vi "ShooterB Test.vi"(0 "Shooter":dbl, 1 "Encoder":dbl, 2 "GetMotorOut":dbl) -> (3 "ToMotor":dbl, 4 "EncoderRPS 2":dbl, 5 "CurentSpeed":dbl, 6 "SpeedWanted":dbl)   [LabVIEW 2011]
uses:
  RobotBetImunim/Robot Global Data.vi
panel:
  out "Waveform Chart 2":dbl(graph)
  out "Waveform Chart":dbl(graph)
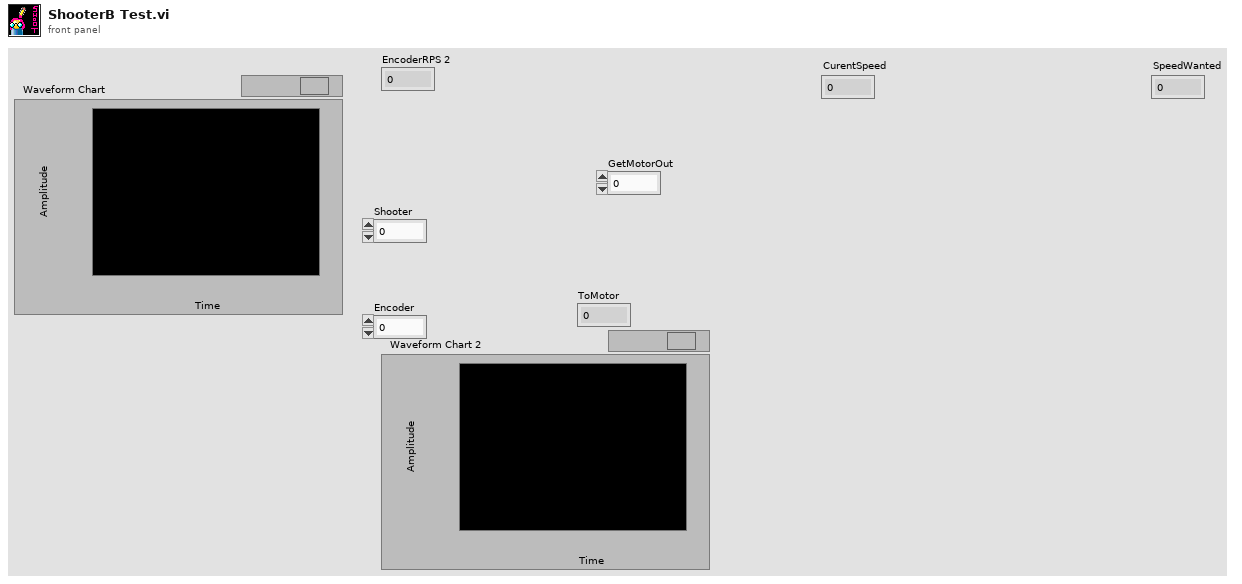
[diagram p1: front panel]
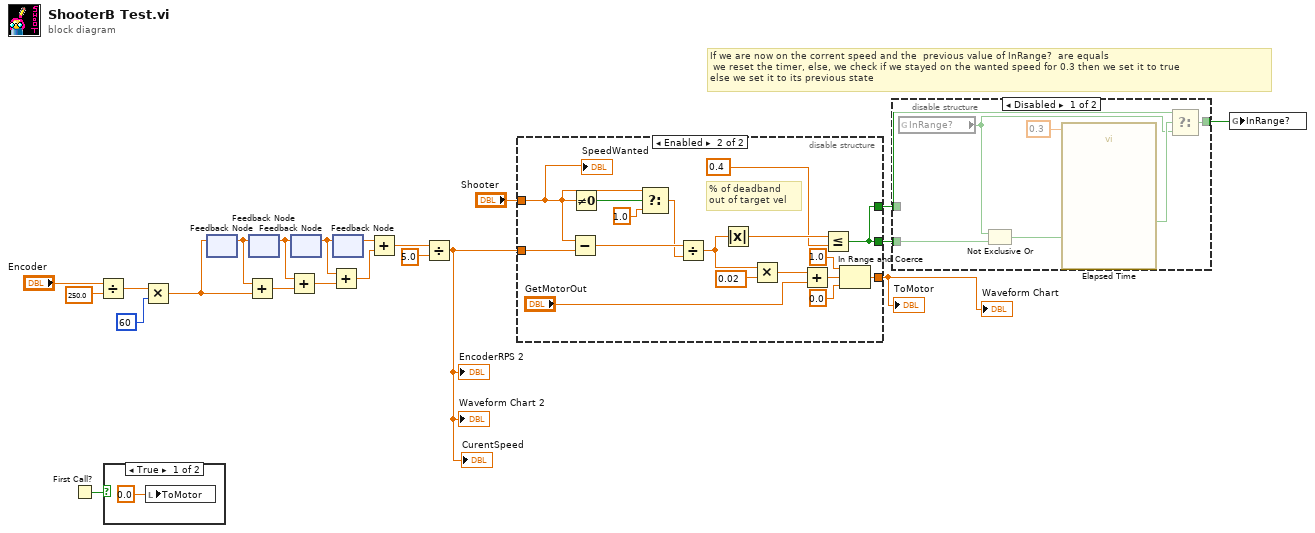
[diagram p0: block diagram]
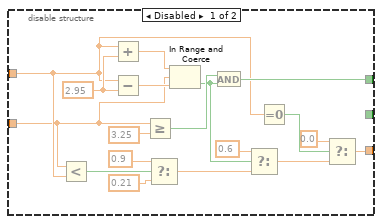
[diagram p4: hidden frame]
diagram:
  # "If we are now on the corrent speed and the  previous value of InRange?  are equals\n we reset the timer, else, we check if we stayed on the wanted speed for 0.3 then we set it to true\nelse we set it to its previous state"
  n1 = First Call?() -> (First Call?: T/F=w8:bool)
  n2 = Divide(x="Encoder", y=250.0) -> (x/y=w4:dbl)
  n3 = case shown="True" w8 {
    frame True {
      n4 = local write "ToMotor"(0.0 ("ToMotor")) -> ()
    }
    frame False {
    }
  }
  n5 = Multiply(x=w4, y=60) -> (x*y=w3:dbl)
  n6 = feedback #1() -> (w14:dbl)  [unwired: 1 in]
  n7 = feedback-in #1(w3) -> ()
  n8 = Add(x=w14, y=w3) -> (x+y=w13:dbl)
  n9 = feedback #2() -> (w18:dbl)  [unwired: 1 in]
  n10 = feedback-in #2(w14) -> ()
  n11 = Add(x=w18, y=w13) -> (x+y=w19:dbl)
  n12 = feedback #3() -> (w16:dbl)  [unwired: 1 in]
  n13 = feedback-in #3(w18) -> ()
  n14 = Add(x=w16, y=w19) -> (x+y=w17:dbl)
  n15 = feedback #4() -> (w15:dbl)  [unwired: 1 in]
  n16 = feedback-in #4(w16) -> ()
  n17 = Add(x=w15, y=w17) -> (x+y=w20:dbl)
  n18 = Divide(x=w20, y=5.0) -> (x/y=w1:dbl)
  "EncoderRPS 2" <- w1
  "Waveform Chart 2" <- w1
  "CurentSpeed" <- w1
  n19 = disable-structure shown="Enabled" {
    disable-tunnel: [w30 w44] -> w10
    disable-tunnel: [w27 w46] -> w6
    disable-tunnel: "Shooter" -> [w24 w41]
    disable-tunnel: w1 -> [w23 w57]
    disable-tunnel: [_ w46] -> w7
    frame Disabled {
      w39 = 2.95
      n20 = Less?(x=w23, y=w24) -> (x < y?=w25:bool)
      n21 = Add(x=w24, y=w39) -> (x+y=w38:dbl)
      n22 = Subtract(x=w24, y=w39) -> (x-y=w37:dbl)
      n23 = Greater Or Equal?(x=w23, y=3.25) -> (x >= y?=w28:bool)
      n24 = Select(t=0.9, s=w25, f=0.21) -> (s? t:f=w35:dbl)
      n25 = In Range and Coerce(upper limit=w38, x=w23, lower limit=w37) -> (In Range?=w26:bool)  [unwired: 1 out]
      n26 = And(x=w28, y=w26) -> (x .and. y?=w27:bool)
      n27 = Select(t=0.6, s=w26, f=w35) -> (s? t:f=w32:dbl)
      n28 = Equal To 0?(x=w24) -> (x = 0?=w31:bool)
      n29 = Select(t=0.0, s=w31, f=w32) -> (s? t:f=w30:dbl)
    }
    frame Enabled {
      # "% of deadband\nout of target vel"
      n30 = Subtract(x=w41, y=w57) -> (x-y=w54:dbl)
      n31 = Not Equal To 0?(x=w41) -> (x != 0?=w52:bool)
      n32 = Select(t=w41, s=w52, f=1.0) -> (s? t:f=w51:dbl)
      n33 = Divide(x=w54, y=w51) -> (x/y=w49:dbl)
      n34 = Absolute Value(x=w49) -> (abs(x)=w48:dbl)
      n35 = Multiply(x=w49, y=0.02) -> (x*y=w53:dbl)
      n36 = Add(x=w53, y="GetMotorOut") -> (x+y=w55:dbl)
      n37 = Less Or Equal?(x=w48, y=0.4) -> (x <= y?=w46:bool)
      n38 = In Range and Coerce(upper limit=1.0, x=w55, lower limit=0.0) -> (coerced(x)=w44:dbl)  [unwired: 1 out]
      "SpeedWanted" <- w41
    }
  }
  "ToMotor" <- w10
  "Waveform Chart" <- w10
  n39 = disable-structure shown="Disabled" {
    disable-tunnel: w7 -> [w64 _]
    disable-tunnel: w6 -> [w60 w65]
    disable-tunnel: [w59 w65] -> w5
    frame Disabled {
      n40 = global read "Robot Global Data.vi" "InRange?"() -> (w58:bool)
      n41 = Not Exclusive Or(1:w64, 2:w58) -> (0:w63:bool)
      n42 = call "Elapsed Time"("Time Target (s)"=0.3, "Reset"=w63) -> ("Time has Elapsed"=w61:bool)  [unwired: 10 in, 7 out]
      n43 = Select(t=w60, s=w61, f=w58) -> (s? t:f=w59:bool)
    }
    frame Enabled {
    }
  }
  n44 = global write "Robot Global Data.vi" "InRange?"(w5) -> ()
